vi "Read write sensor info.vi"(8 "error in (no error)":errorcluster, 10 "Table Control in":string[][](table), 11 "Read/Write":u16(ring) items=["READ", "WRITE"]) -> (0 "error out":errorcluster, 3 "Table Control out":string[][](table))   [LabVIEW 2015]
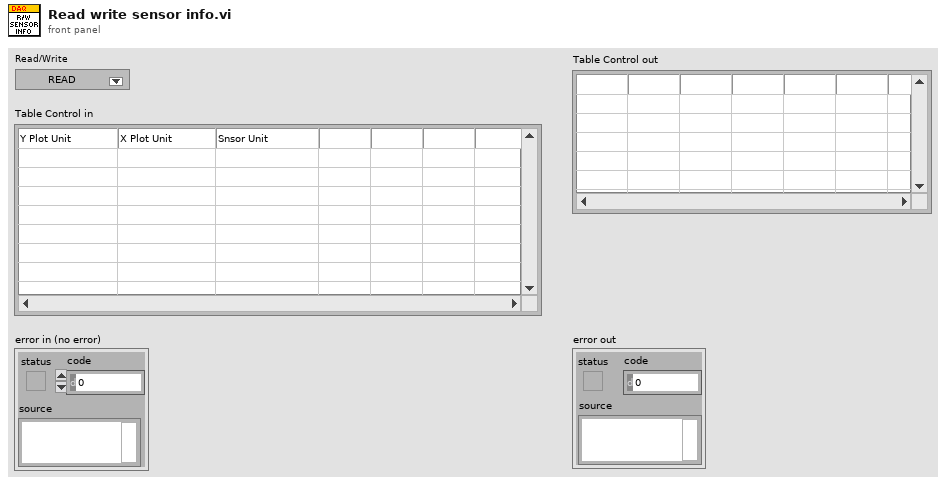
[diagram p1: front panel]
types:
  T1 = enum16{"open", "replace", "create", "open or create", "replace or create", "replace or create with confirmation"}
  T2 = enum16{"read/write", "read-only", "write-only", "write-only (truncate)"}
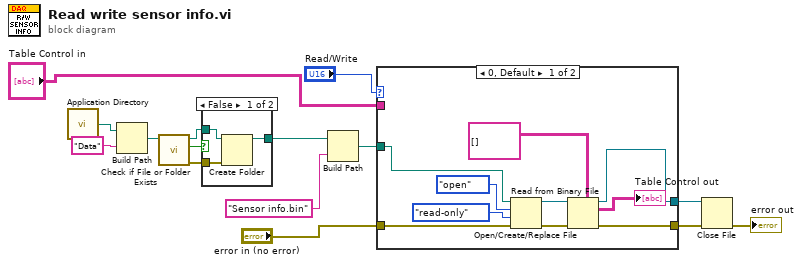
[diagram p0: block diagram]
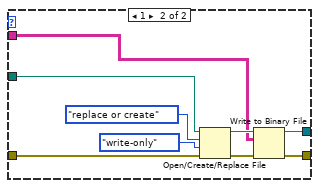
[diagram p3: hidden frame]
diagram:
  n1 = call <vilib>:"Application Directory.vi"() -> ("Application Directory"=w10:path)
  n2 = Build Path(base path=w10, name or relative path="Data") -> (appended path=w6:path)
  n3 = call <vilib>:"Check if File or Folder Exists.vi"("path"=w6) -> ("error out"=w4:errorcluster, "file or folder exists?"=w5:bool, "dup path"=w3:path)  [unwired: 8 in]
  n4 = case shown="False" w5 {
    tunnel: w4 -> [w18 _]
    tunnel: w3 -> [w17 w19]
    tunnel: [w16 w19] -> w2
    frame False {
      n5 = Create Folder(path (use dialog)=w17, error in=w18) -> (created path=w16:path)  [unwired: 1 in, 2 out]
    }
    frame True {
    }
  }
  n6 = Build Path(base path=w2, name or relative path="Sensor info.bin") -> (appended path=w7:path)
  n7 = case shown="0, Default" "Read/Write" {
    tunnel: [w27 w36] -> w14
    tunnel: [w26 w35] -> w13
    tunnel: w7 -> [w25 w38]
    tunnel: "error in (no error)" -> [w24 w37]
    tunnel: "Table Control in" -> [_ w30]
    frame 0, Default {
      n8 = Open/Create/Replace File(file path (use dialog)=w25, error in=w24, operation (0:open)=T1."open", access (0:read/write)=T2."read-only" ("open mode (0)")) -> (refnum out=w29:refnum<file>, error out=w28:errorcluster)  [unwired: 2 in, 1 out]
      n9 = Read from Binary File(5:string[][] [] ("Table Control 3"), 8:w28, 11:w29) -> (0:w26:errorcluster, 2:→"Table Control out":string[][], 3:w27:refnum<file>)  [unwired: 4 out]
    }
    frame 1 {
      n10 = Open/Create/Replace File(file path (use dialog)=w38, error in=w37, operation (0:open)=T1."replace or create", access (0:read/write)=enum16{"read/write", "read-only", "write-only"}."write-only") -> (refnum out=w34:refnum<file>, error out=w33:errorcluster)  [unwired: 2 in, 1 out]
      n11 = Write to Binary File(file (use dialog)=w34, data=w30, error in=w33) -> (refnum out=w36:refnum<file>, error out=w35:errorcluster)  [unwired: 4 out]
    }
  }
  n12 = Close File(refnum=w14, error in=w13) -> (error out=→"error out":errorcluster)  [unwired: 1 out]
